vi "仁科空调控制器告警存储.vi"(11 "x+1":refnum<vi>) -> ()   [LabVIEW 2016, in "环境动力监测库.lvlib" / "空调库.lvlib"]
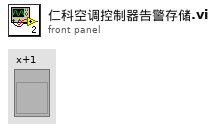
[diagram p1: front panel]
types:
  T1 = cluster{"型号选择":enum16{"黑盾", "英维克", "仁科测控RS-KTC-N01"}, "MB session in":refnum<class "MB_Master.lvclass">, "英维克空调寄存器":u16[], "通讯状态":bool, "PORT":string, "IP":string, "Slave ID ":u8, "Serial Config":cluster{"baud rate (bps)":u32, "stop bits":u16, "parity":u16, "flow control":u16, "timeout":u32, "retries":i32}, "VISA Resource":refnum<visa-resource-name>, "MB通信方式选择":enum16{"串口", "TCP"}, "系统参数":cluster{"空调开启点":u16, "空调灵敏点":u16, "加热开启点":u16, "加热灵敏度":u16, "高温告警点":u16, "低温告警点":u16}}
  T2 = cluster{"温湿度解析":cluster{"湿度":dbl, "温度":dbl}, "传感器状态输出":cluster{"第一路电流A":u16, "第二路电流A":u16, "空调控制模式":enum16{"远程", "自动"}, "蜂鸣器和继电器报警输出状态":enum16{"正常", "报警"}, "秒数高16位":u16, "秒数低16位":u16}, "告警状态":cluster{"第一路开关机失败":bool, "第二路开关机失败":bool, "温度超上限报警":bool, "温度超下限报警":bool}, "运行状态":cluster{"第一路空调运行状态":enum16{"停止", "制冷", "制热", "未知"}, "第二路空调运行状态":enum16{"停止", "制冷", "制热", "未知"}}}
  T3 = cluster{"漏水监测输出":cluster{"漏水监测告警":bool, "告警内容":string}, "门禁监测输出":cluster{"门禁监测告警":bool, "告警内容":string}, "门禁监测输出2":cluster{"门禁监测告警":bool, "告警内容":string}, "温湿度监测输出":cluster{"温湿度监测告警":bool, "告警内容":string}, "烟雾监测输出":cluster{"烟雾监测告警":bool, "告警内容":string}, "空调监测输出":cluster{"空调监测告警":bool, "告警内容":string}, "自动重合闸输出":cluster{"自动重合闸告警":bool, "告警内容":string}, "红外入侵输出":cluster{"红外入侵告警":bool, "告警内容":string}, "振动输出":cluster{"振动告警":bool, "告警内容":string}, "UPS输出":cluster{"UPS告警":bool, "告警内容":string}, "蓄电池输出":cluster{"蓄电池告警":bool, "告警内容":string}, "蓄电池输出2":cluster{"蓄电池告警":bool, "告警内容":string}, "GPS输出":cluster{"定位告警":bool, "告警内容":string}, "北斗输出":cluster{"定位告警":bool, "告警内容":string}, "气象输出":cluster{"气象告警":bool, "告警内容":string}, "废液输出":cluster{"废液告警":bool, "告警内容":string}, "废液输出2":cluster{"废液告警":bool, "告警内容":string}}
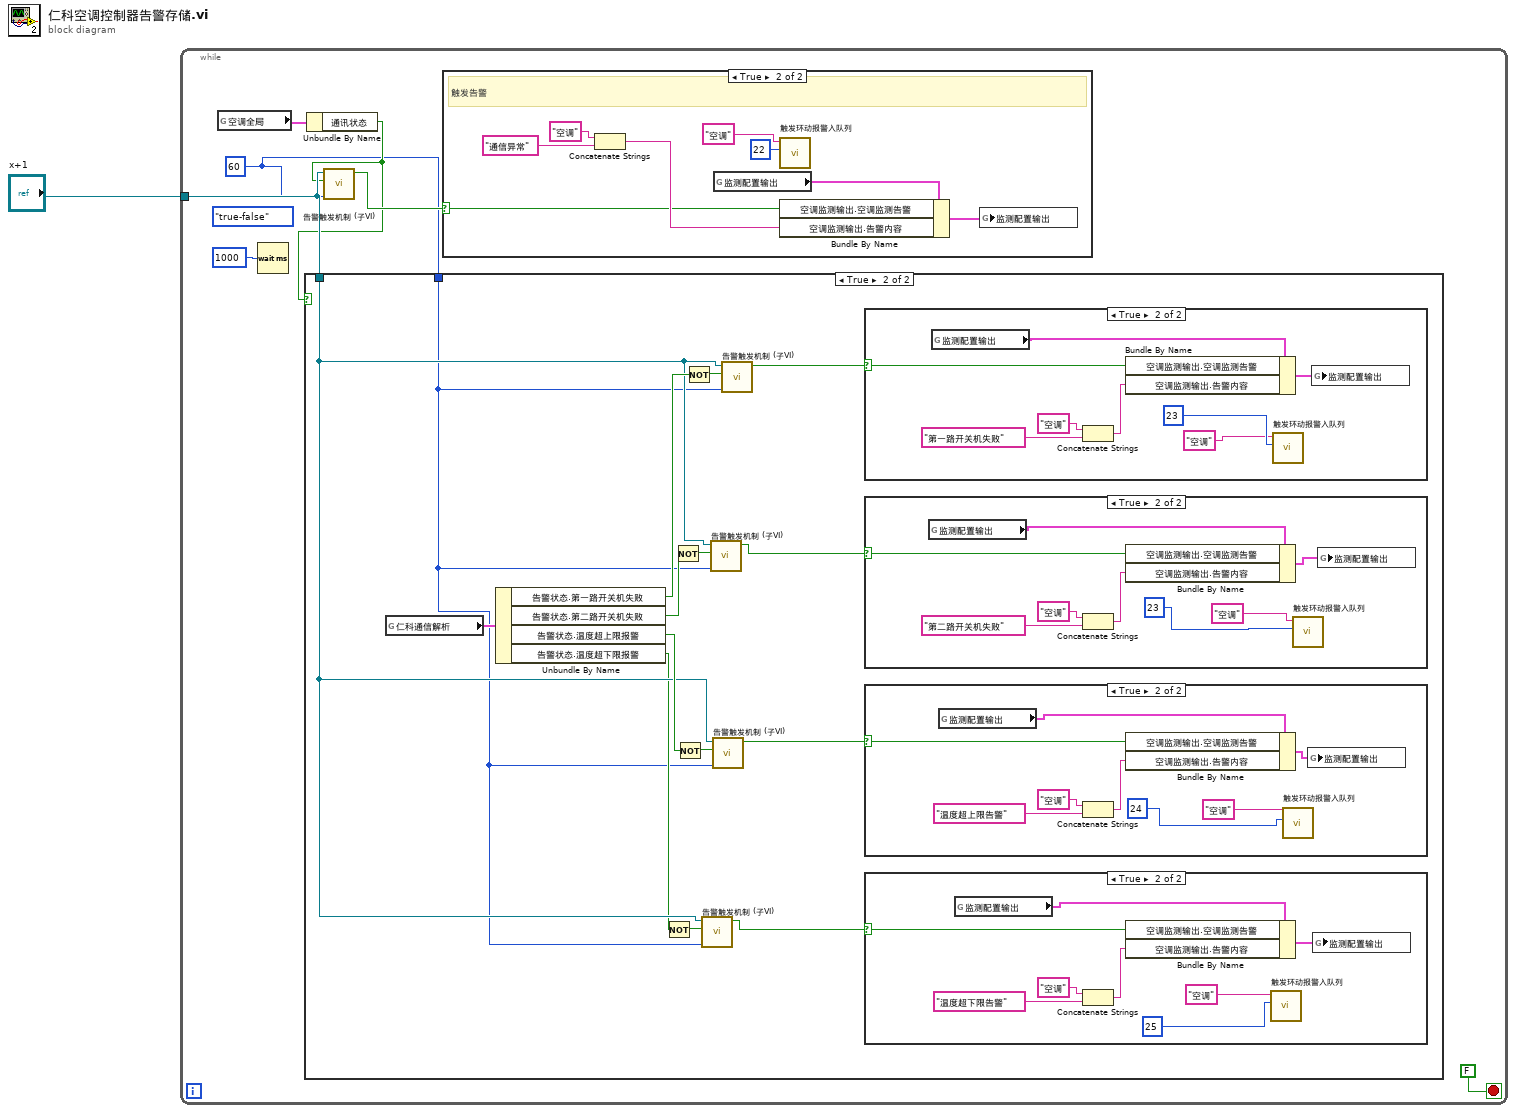
[diagram p0: block diagram]
diagram:
  n1 = while {
    tunnel: "x+1" -> [w5]
    stop <- FALSE stop-if-true
    w2 = u32 60 ("信号持续时间")
    (unwired) enum16{"either", "false-true", "true-false"}."true-false" ("direction")
    n2 = global read "断电保存全局变量.vi" "空调全局"() -> (w4:T1)
    n3 = Wait (ms)(milliseconds to wait=u32 1000 ("等待时间（毫秒）")) -> ()  [unwired: 1 out]
    n4 = Unbundle By Name(w4) -> ("通讯状态"=w3:bool)
    n5 = case shown="True" w3 {
      tunnel: w5 -> [_ w12]
      tunnel: w2 -> [_ w9]
      frame False {
      }
      frame True {
        n6 = global read "内部交互全局变量.vi" "仁科通信解析"() -> (w23:T2)
        n7 = Unbundle By Name(w23) -> ("告警状态.第一路开关机失败"=w20:bool, "告警状态.第二路开关机失败"=w17:bool, "告警状态.温度超上限报警"=w13:bool, "告警状态.温度超下限报警"=w11:bool)
        n8 = Not(x=w11) -> (.not. x?=w16:bool)
        n9 = Not(x=w17) -> (.not. x?=w19:bool)
        n10 = Not(x=w13) -> (.not. x?=w15:bool)
        n11 = Not(x=w20) -> (.not. x?=w22:bool)
        n12 = call "告警触发机制 (子VI).vi"("信号持续时间"=w9, "状态输出真-正常"=w16, "Digital输入"=w12) -> ("触发告警"=w10:bool)  [unwired: 6 in, 2 out]
        n13 = call "告警触发机制 (子VI).vi"("信号持续时间"=w9, "状态输出真-正常"=w19, "Digital输入"=w12) -> ("触发告警"=w18:bool)  [unwired: 6 in, 2 out]
        n14 = call "告警触发机制 (子VI).vi"("信号持续时间"=w9, "状态输出真-正常"=w15, "Digital输入"=w12) -> ("触发告警"=w14:bool)  [unwired: 6 in, 2 out]
        n15 = call "告警触发机制 (子VI).vi"("信号持续时间"=w9, "状态输出真-正常"=w22, "Digital输入"=w12) -> ("触发告警"=w21:bool)  [unwired: 6 in, 2 out]
        n16 = case shown="True" w21 {
          selector: w21 -> [_ w47]
          frame False {
          }
          frame True {
            n17 = global read "内部交互全局变量.vi" "监测配置输出"() -> (w44:T3)
            n18 = Concatenate Strings("空调" ("设备"), "第一路开关机失败" ("日志信息")) -> (w45:string)
            n19 = Bundle By Name(cluster=w44, "空调监测输出.空调监测告警"=w47, "空调监测输出.告警内容"=w45) -> (w43:T3)
            n20 = call "触发环动报警入队列.vi"("code"=23, "元器件"="空调" ("设备")) -> ()  [unwired: 10 in]
            n21 = global write "内部交互全局变量.vi" "监测配置输出"(w43) -> ()
          }
        }
        n22 = case shown="True" w18 {
          selector: w18 -> [_ w39]
          frame False {
          }
          frame True {
            n23 = global read "内部交互全局变量.vi" "监测配置输出"() -> (w36:T3)
            n24 = Concatenate Strings("空调" ("设备"), "第二路开关机失败" ("日志信息")) -> (w37:string)
            n25 = Bundle By Name(cluster=w36, "空调监测输出.空调监测告警"=w39, "空调监测输出.告警内容"=w37) -> (w35:T3)
            n26 = call "触发环动报警入队列.vi"("code"=23, "元器件"="空调" ("设备")) -> ()  [unwired: 10 in]
            n27 = global write "内部交互全局变量.vi" "监测配置输出"(w35) -> ()
          }
        }
        n28 = case shown="True" w14 {
          selector: w14 -> [_ w55]
          frame False {
          }
          frame True {
            n29 = global read "内部交互全局变量.vi" "监测配置输出"() -> (w52:T3)
            n30 = Concatenate Strings("空调" ("设备"), "温度超上限告警" ("日志信息")) -> (w53:string)
            n31 = Bundle By Name(cluster=w52, "空调监测输出.空调监测告警"=w55, "空调监测输出.告警内容"=w53) -> (w51:T3)
            n32 = call "触发环动报警入队列.vi"("code"=24, "元器件"="空调" ("设备")) -> ()  [unwired: 10 in]
            n33 = global write "内部交互全局变量.vi" "监测配置输出"(w51) -> ()
          }
        }
        n34 = case shown="True" w10 {
          selector: w10 -> [_ w31]
          frame False {
          }
          frame True {
            n35 = global read "内部交互全局变量.vi" "监测配置输出"() -> (w28:T3)
            n36 = Concatenate Strings("空调" ("设备"), "温度超下限告警" ("日志信息")) -> (w29:string)
            n37 = Bundle By Name(cluster=w28, "空调监测输出.空调监测告警"=w31, "空调监测输出.告警内容"=w29) -> (w27:T3)
            n38 = call "触发环动报警入队列.vi"("code"=25, "元器件"="空调" ("设备")) -> ()  [unwired: 10 in]
            n39 = global write "内部交互全局变量.vi" "监测配置输出"(w27) -> ()
          }
        }
      }
    }
    n40 = call "告警触发机制 (子VI).vi"("信号持续时间"=w2, "状态输出真-正常"=w3, "Digital输入"=w5) -> ("触发告警"=w6:bool)  [unwired: 6 in, 2 out]
    n41 = case shown="True" w6 {
      selector: w6 -> [_ w61]
      frame False {
      }
      frame True {
        # "触发告警"
        n42 = Concatenate Strings("空调" ("设备"), "通信异常" ("日志信息")) -> (w62:string)
        n43 = global read "内部交互全局变量.vi" "监测配置输出"() -> (w60:T3)
        n44 = call "触发环动报警入队列.vi"("code"=22, "元器件"="空调" ("设备")) -> ()  [unwired: 10 in]
        n45 = Bundle By Name(cluster=w60, "空调监测输出.空调监测告警"=w61, "空调监测输出.告警内容"=w62) -> (w59:T3)
        n46 = global write "内部交互全局变量.vi" "监测配置输出"(w59) -> ()
      }
    }
  }
